vi "Read file.vi"(8 "error in (no error)":errorcluster, 11 "Ephemeris in":refnum<class "Ephemeris.lvclass">) -> (0 "error out":errorcluster, 2 "file":string, 3 "Ephemeris out":refnum<class "Ephemeris.lvclass">)   [LabVIEW 2022 SP3, in "TCSDataDefinitions.lvlib" / "TCSCommand.lvlib" / "TargetConfiguration.lvlib" / "Target.lvlib" / "Ephemeris.lvclass"]
uses:
  Ephemeris.lvclass
  Ephemeris.lvclass/Ephemeris.ctl
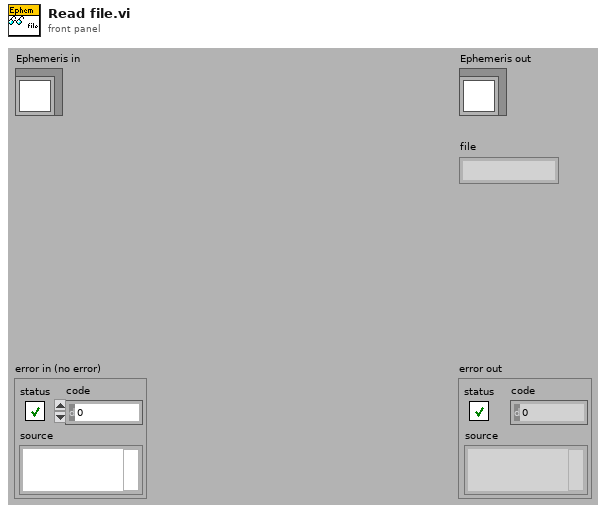
[diagram p1: front panel]
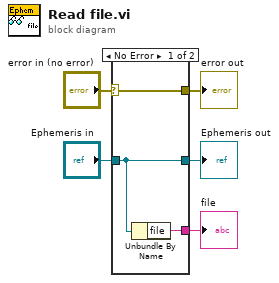
[diagram p0: block diagram]
diagram:
  n1 = case shown="No Error" "error in (no error)" {
    selector: "error in (no error)" -> [w8 w9]
    tunnel: [w8 w9] -> w4
    tunnel: [w7 w10] -> w2
    tunnel: "Ephemeris in" -> [w7 w10]
    tunnel: [w6 _] -> w1
    frame No Error {
      n2 = Unbundle By Name(w7) -> ("file"=w6:string)
    }
    frame Error {
    }
  }
  "error out" <- w4
  "Ephemeris out" <- w2
  "file" <- w1
